vi "LEBITplc.PubLastLoadedFileServices.vi"(0 "i ref in":refnum<vi>, 2 "i attribute in":T1, 5 "error in":errorcluster) -> (14 "i ref out":refnum<vi>, 16 "i attribute out":T1, 17 "GUIServiceID":i32[](array[numeric]), 19 "error out":errorcluster)   [LabVIEW 2014, in "LEBITplc.lvlib"]
uses:
  LEBITplc.lvlib
  LEBITplc.i attribute.ctl
  CSlibraries/UtilityLib/UtilityLib.valueStatus.ctl
  CSlibraries/UtilityLib/UtilityLib.lvlib
  CS_Core/CSSystem/CoreLib/CoreLib.lvlib
  CSlibraries-extern/DimLVEvent/LVDimInterface/LVDimInterface.lvlib
  TestPanel/Panels.lvlib
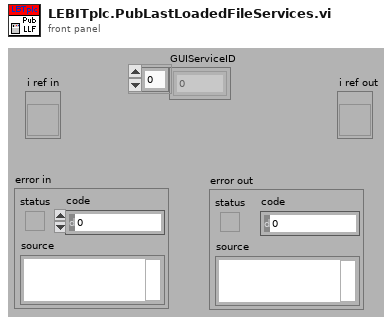
[diagram p1: front panel]
types:
  T1 = typedef "LEBITplc.lvlib/LEBITplc.i attribute.ctl" = cluster{"LLFLocation":string, "SetFileLocation":string, "nickNames":string[], "setValuePLCServiceID":i32[], "GUIServiceID":i32[], "monValuePLC":string[], "SetValueServiceID":i32[], "MonValueServiceID":i32[], "SetValue":dbl[][], "SetValueMin":dbl[], "SetValueMax":dbl[], "SetValueInfoServiceID":i32[], "GUINames":string[], "ListOfBases":string[], "Scale":dbl[], "Offset":dbl[], "setValuePLC":string[], "BaseName":string[], "ScaleServiceID":i32[], "OffsetServiceID":i32[], "AllPLCValues":string[], "CondSpecialArray":string[][], "CondSpecialIndex":i32[], "CondSpecialMonValue":dbl[], "RecentlyChanged":i32[], "SetFileLocationID":i32, "Dependent-Monitors":string[][], "LastLoadedFiles":string[], "IonGuideCalibLocation":string, "Monitor Dependent":string[], "Special":string[], "PLC?":bool[], "Start Date":string, "ListOfBasesServiceID":i32, "SETRA VISA resource":refnum<visa-resource-name>}
  T2 = typedef "UtilityLib.lvlib/UtilityLib.valueStatus.ctl" = enum16{"no info available", "stand by/off", "on", "warning", "alarm/malfunction", "not implemented", "user action required", "important information", "system default", "control default", "indicator default", "button default"}
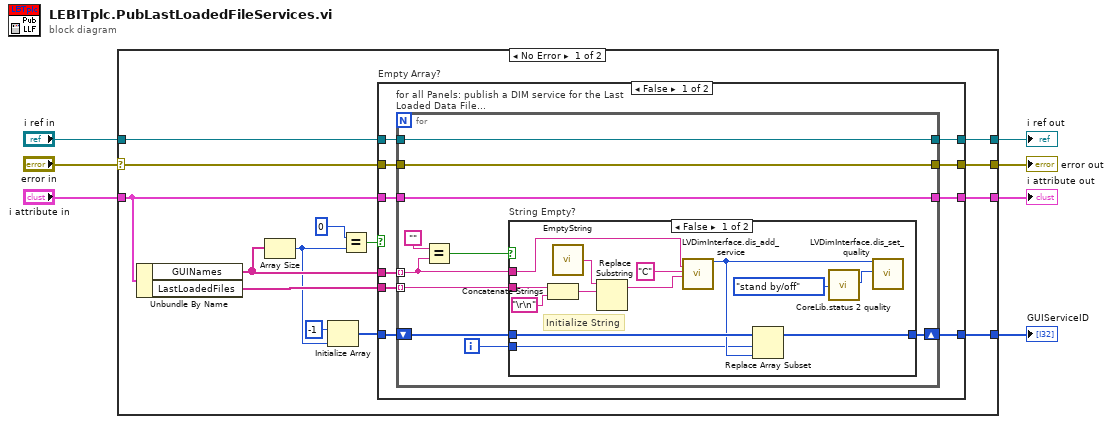
[diagram p0: block diagram]
diagram:
  n1 = case shown="No Error" "error in" {
    selector: "error in" -> [w17 w61]
    tunnel: "i attribute in" -> [w16 w60]
    tunnel: [w21 w61] -> w6
    tunnel: [w20 w62] -> w5
    tunnel: "i ref in" -> [w19 w62]
    tunnel: [w18 _] -> w3
    tunnel: [w15 w60] -> w1
    frame No Error {
      n2 = Unbundle By Name(w16) -> ("GUINames"=w12:string[], "LastLoadedFiles"=w11:string[])
      n3 = Array Size(array=w12) -> (size(s)=w9:i32)
      n4 = Initialize Array(-1 ("x"), w9) -> (w10:i32[])
      n5 = Equal?(x=0, y=w9) -> (x = y?=w14:bool)
      n6 = case "Empty Array?" shown="False" w14 {
        tunnel: [w31 w58] -> w21
        tunnel: [w30 w59] -> w20
        tunnel: w19 -> [w29 w59]
        tunnel: w10 -> [w28 w56]
        tunnel: [w27 w56] -> w18
        tunnel: w17 -> [w26 w58]
        tunnel: w16 -> [w25 w57]
        tunnel: [w24 w57] -> w15
        tunnel: w12 -> [w23 _]
        tunnel: w11 -> [w22 _]
        frame False {
          n7 = for "for all Panels: publish a DIM service for the Last Loaded Data File..." {
            tunnel: w29 -> [w40]
            tunnel: w26 -> [w39]
            tunnel: [w39] -> w31
            tunnel: [w40] -> w30
            shift-right: [w38] -> w27
            shift-left: w28 -> [w41]
            tunnel: w23 -> [w35] mode=indexing
            tunnel: w25 -> [w37]
            tunnel: [w37] -> w24
            tunnel: w22 -> [w34] mode=indexing
            i -> [w36]
            n8 = Equal?(x="", y=w35) -> (x = y?=w32:bool)
            n9 = case "String Empty?" shown="False" w32 {
              tunnel: w41 -> [w54 w55]
              tunnel: [w53 w55] -> w38
              tunnel: w34 -> [w45 _]
              tunnel: w35 -> [w43 _]
              tunnel: w36 -> [w42 _]
              frame False {
                # "Initialize String"
                n10 = Concatenate Strings(w45, "\r\n") -> (w46:string)
                n11 = call "EmptyString.vi"() -> ("String"=w48:string)
                n12 = Replace Substring(4:w46, 5:w48) -> (1:w44:string)  [unwired: 2 in, 1 out]
                n13 = call "LVDimInterface.dis_add_service.vi"("serviceName"=w43, "typeDescriptor"="C", "data"=w44) -> ("my_serviceID"=w50:i32)  [unwired: 15 in, 1 out]
                n14 = Replace Array Subset(array=w54, new element=w50, index=w42) -> (w53:i32[])
                n15 = call "CoreLib.status 2 quality.vi"("valueStatus"=UtilityLib.valueStatus."stand by/off") -> ("quality"=w52:i32)  [unwired: 18 in]
                n16 = call "LVDimInterface.dis_set_quality.vi"("my_serviceID"=w50, "quality"=w52) -> ()  [unwired: 16 in, 2 out]
              }
              frame True {
              }
            }
          }
        }
        frame True {
        }
      }
    }
    frame Error {
    }
  }
  "error out" <- w6
  "i ref out" <- w5
  "GUIServiceID" <- w3
  "i attribute out" <- w1
